vi "sweep_from_Zero.vi"(4 "Forward/Reverse":bool, 5 "Point Number":i32, 6 "Step Size":dbl format="%.2f", 7 "Sweep Stop":dbl format="%.2f", 8 "Sweep Start":dbl format="%.2f") -> (1 "Active":bool, 3 "Output":dbl format="%.2f")   [LabVIEW 2017]
panel:
  out "Array":dbl[](array[numeric])
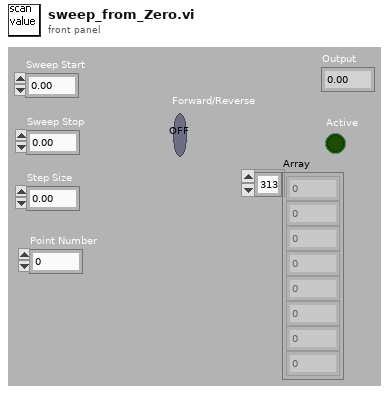
[diagram p1: front panel]
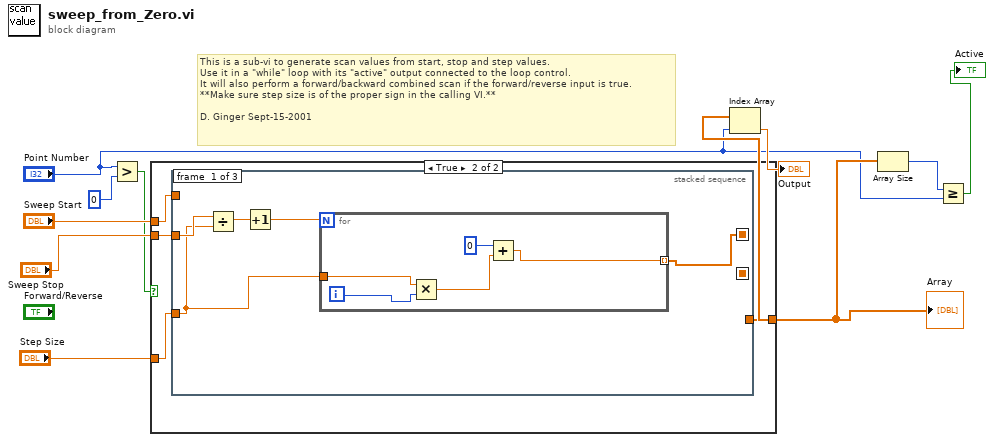
[diagram p0: block diagram]
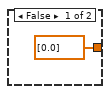
[diagram p2: hidden frame]
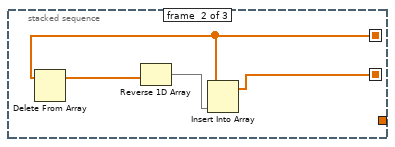
[diagram p3: hidden frame]
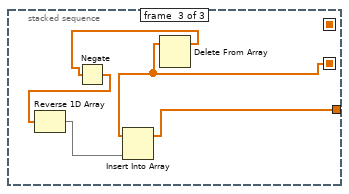
[diagram p4: hidden frame]
diagram:
  # "This is a sub-vi to generate scan values from start, stop and step values.\nUse it in a \"while\" loop with its \"active\" output connected to the loop control.\nIt will also perform a forward/backward combined scan if the forward/reverse input is true.\n**Make sure step size is of the proper sign in the calling VI.**\n\nD. Ginger Sept-15-2001"
  n1 = Greater?(x="Point Number", y=0) -> (0:w5:bool)
  n2 = case shown="True" w5 {
    tunnel: "Sweep Start" -> [_ w15]
    tunnel: "Sweep Stop" -> [_ w14]
    tunnel: "Step Size" -> [_ w13]
    tunnel: [dbl[] [0.0] w12] -> w4
    frame False {
    }
    frame True {
      n3 = stacked-sequence {
        seq-local: [w17 _ _] -> [_ w27 _]
        seq-local: [_ w28 _] -> [_ _ w30]
        tunnel: w15 -> [_ _ _]
        tunnel: w14 -> [w20 _ _]
        tunnel: w13 -> [w19 _ _]
        tunnel: [_ _ w33] -> w12
        frame #0 {
          n4 = Divide(x=w20, y=w19) -> (x/y=w18:dbl)
          n5 = Increment(x=w18) -> (x+1=w16:dbl)
          n6 = for {
            N: w16 -> [_]
            tunnel: [w25] -> w17 mode=indexing
            tunnel: w19 -> [w22]
            i -> [w21]
            n7 = Multiply(x=w22, y=w21) -> (x*y=w24:dbl)
            n8 = Add(x=0, y=w24) -> (x+y=w25:dbl)
          }
        }
        frame #1 {
          n9 = Delete From Array(array=w27) -> (array with subset deleted=w26:dbl[])  [unwired: 2 in, 1 out]
          n10 = Reverse 1D Array(array=w26) -> (reversed array=w29:dbl[])
          n11 = Insert Into Array(array=w27, new element=w29) -> (w28:dbl[])  [unwired: 1 in]
        }
        frame #2 {
          n12 = Delete From Array(array=w30) -> (array with subset deleted=w32:dbl[])  [unwired: 2 in, 1 out]
          n13 = Negate(x=w32) -> (-x=w31:dbl[])
          n14 = Reverse 1D Array(array=w31) -> (reversed array=w34:dbl[])
          n15 = Insert Into Array(array=w30, new element=w34) -> (w33:dbl[])  [unwired: 1 in]
        }
      }
    }
  }
  "Array" <- w4
  n16 = Index Array(array=w4, index="Point Number") -> (element=→"Output":dbl)
  n17 = Array Size(array=w4) -> (size(s)=w3:i32)
  n18 = Greater Or Equal?(x=w3, y="Point Number") -> (x >= y?=→"Active":bool)
